vi "Read state.vi"(11 "Model in":refnum<class "Model.lvclass">) -> (2 "StateValue":T1=enum."OffState", 3 "Model out":refnum<class "Model.lvclass">)   [LabVIEW 2012, in "Model.lvclass"]
uses:
  Model.lvclass
  Typedefs/StateValue.ctl
  Model.lvclass/Model.ctl
  Typedefs/EXATypedefs.lvlib
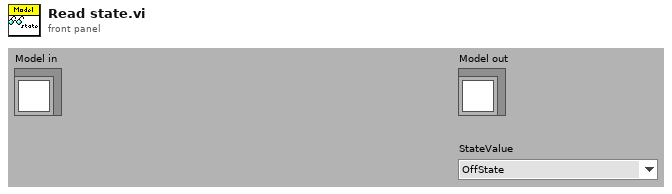
[diagram p1: front panel]
types:
  T1 = typedef "EXATypedefs.lvlib/StateValue.ctl" = enum16{"DisabledState", "EnabledState", "FaultState", "OffState", "StandbyState"}
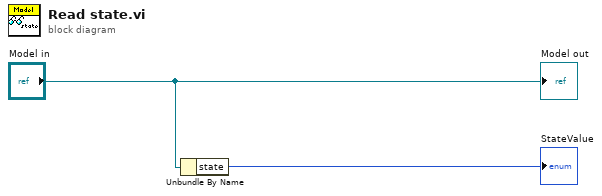
[diagram p0: block diagram]
diagram:
  n1 = Unbundle By Name("Model in") -> ("state"=→"StateValue":T1)
  "Model out" <- "Model in"
